vi "const enable channel name.vi"() -> (3 "enable channel":string)   [LabVIEW 2013, in "Binary datalogger configuration.lvclass"]
uses:
  Binary datalogger configuration.lvclass
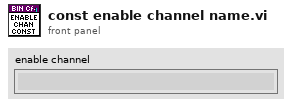
[diagram p1: front panel]
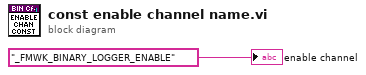
[diagram p0: block diagram]
diagram:
  "enable channel" <- "_FMWK_BINARY_LOGGER_ENABLE" ("enable channel")
